vi "Transmission Dynamics.vi"(9 "Transmission Speed Out (rad/s)":sgl, 10 "Gear":sgl, 11 "Impeller Speed (rad/s)":sgl) -> (1 "Transmission Torque Out (N-m)":sgl, 2 "Impeller Torque (N-m)":sgl)   [LabVIEW 2016, in "NI-PCG Vehicle Model.lvlib"]
uses:
  NI-PCG Vehicle Model.lvlib
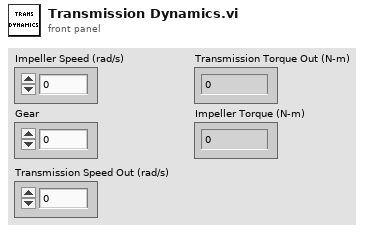
[diagram p1: front panel]
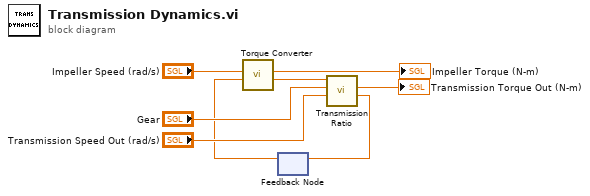
[diagram p0: block diagram]
diagram:
  n1 = feedback #1() -> (w3:sgl)  [unwired: 1 in]
  n2 = call "Torque Converter.vi"("Turbine Speed (rad/s)"=w3, "Impeller Speed (rad/s)"="Impeller Speed (rad/s)") -> ("Turbine Torque (N-m)"=w7:sgl, "Impeller Torque (N-m)"=→"Impeller Torque (N-m)":sgl)  [unwired: 8 in]
  n3 = call "Transmission Ratio.vi"("Transmission Speed Out (rad/s)"="Transmission Speed Out (rad/s)", "Gear"="Gear", "Transmission Torque In (N-m)"=w7) -> ("Transmission Speed In (rad/s)"=w4:sgl, "Transmission Torque Out (N-m)"=→"Transmission Torque Out (N-m)":sgl)  [unwired: 7 in]
  n4 = feedback-in #1(w4) -> ()
